vi "RFID_Barcode_Get.vi"(8 "error in (no error)":errorcluster, 11 "Ref in":T1={"MS SQL Connection"=refnum, "UDL File"=path "", "Time"="", "DCODE"="", "WIP+1"=0, "MC No?"=0, "POKAYOKE?"=FALSE, "Expected Result"="", "Result [Status]"="", "Clock"=0.0, "RFID"="", "WIP Queue"=refnum, "TS Parameter"={"ProfitCenterCode"="", "LineCode"="", "WorkOrderNumber"="", "Model"="", "Model_with_Prefix"="", "VendorCode"="", "SetParameterDateCode"="", "PokaYoke"=0, "Target"=1, "Live_DateCode"="", "CustomerPartNumber"="", "Hand"="", "Ent_Stamp"=timestamp(0 s since 1904-01-01), "STS_CD"=0.0}, "Data_Queue"=[], "RFID Serial No."=""} {"TS Parameter"."Target" min=1 max=100000; "TS Parameter"."PokaYoke" min=0 max=1}) -> (0 "error out":errorcluster, 1 "Serial No":string, 2 "Expected Barcode":string, 3 "Ref out":T1={"MS SQL Connection"=refnum, "UDL File"=path "", "Time"="", "DCODE"="", "WIP+1"=0, "MC No?"=0, "POKAYOKE?"=FALSE, "Expected Result"="", "Result [Status]"="", "Clock"=0.0, "RFID"="", "WIP Queue"=refnum, "TS Parameter"={"ProfitCenterCode"="", "LineCode"="", "WorkOrderNumber"="", "Model"="", "Model_with_Prefix"="", "VendorCode"="", "SetParameterDateCode"="", "PokaYoke"=0, "Target"=1, "Live_DateCode"="", "CustomerPartNumber"="", "Hand"="", "Ent_Stamp"=timestamp(0 s since 1904-01-01), "STS_CD"=0.0}, "Data_Queue"=[], "RFID Serial No."=""} {"TS Parameter"."Target" min=1 max=100000; "TS Parameter"."PokaYoke" min=0 max=1})   [LabVIEW 2020]
uses:
  Controls/TD SQL.ctl
  <vilib>/addons/database/Connection.llb/Conn ObjectReference.ctl
  Controls/WIP_State.ctl
  Controls/TS_Parameter.ctl
  <vilib>/addons/database/NI_Database_API.lvlib
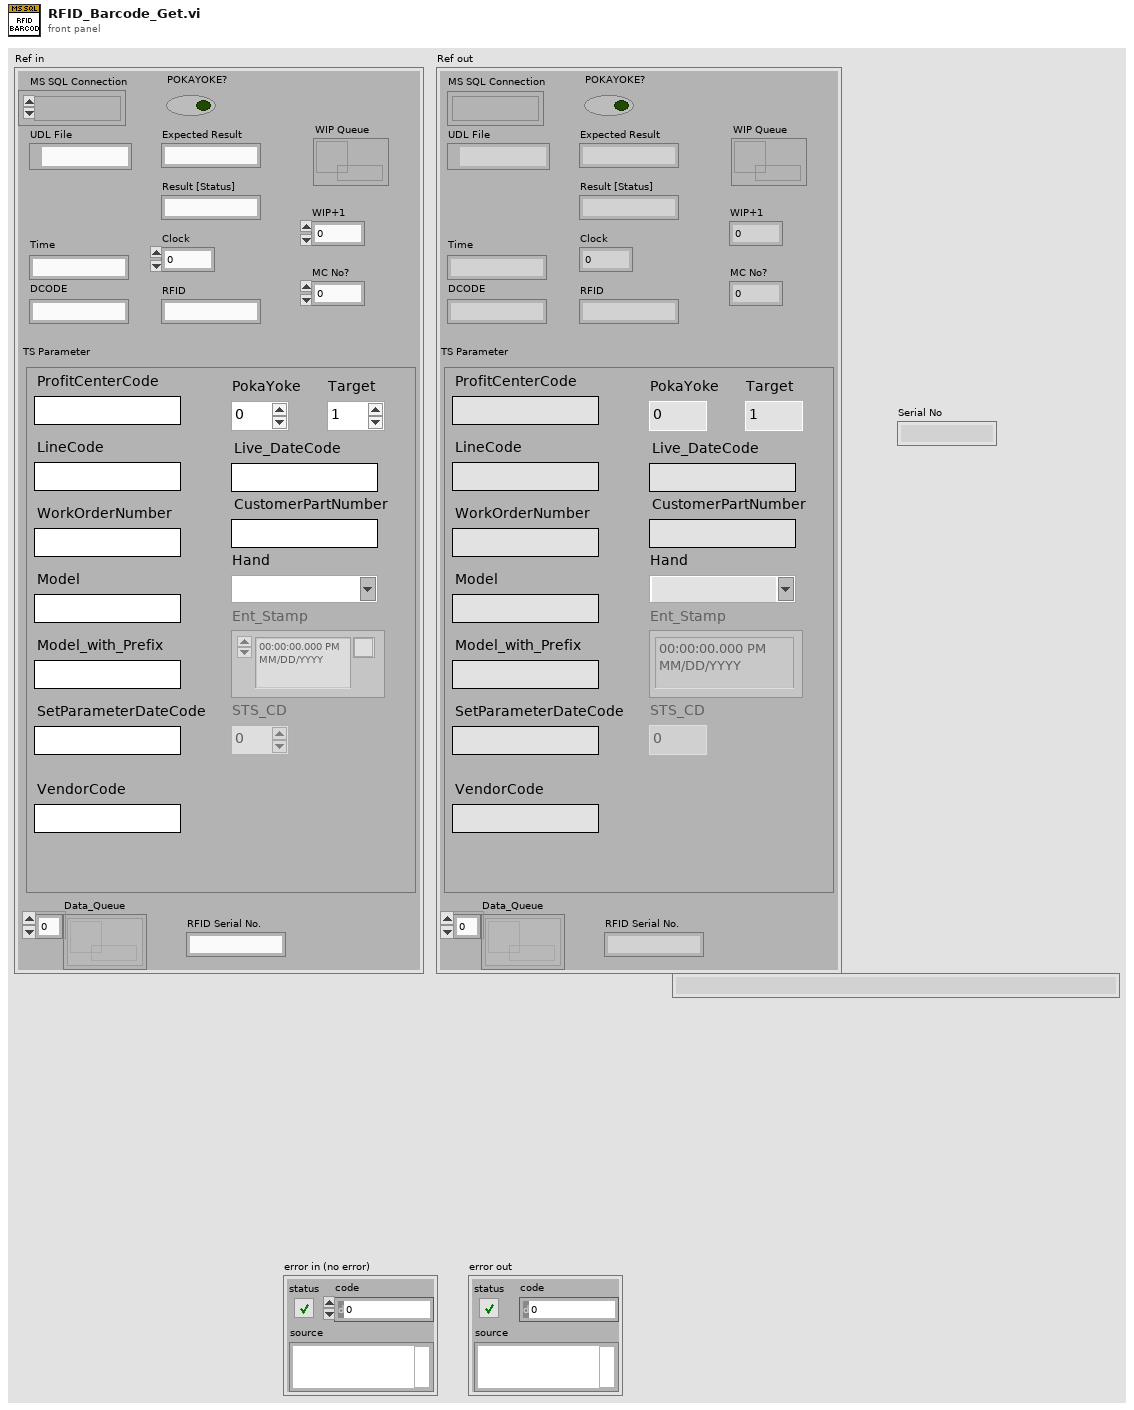
[diagram p1: front panel]
types:
  T1 = typedef "TD SQL.ctl" = cluster{"MS SQL Connection":T2, "UDL File":path, "Time":string, "DCODE":string, "WIP+1":i64, "MC No?":i32, "POKAYOKE?":bool, "Expected Result":string, "Result [Status]":string, "Clock":dbl, "RFID":string, "WIP Queue":refnum<queue>, "TS Parameter":T3, "Data_Queue":refnum<queue>[], "RFID Serial No.":string}
  T2 = typedef "NI_Database_API.lvlib/Conn ObjectReference.ctl" = refnum<k1>
  T3 = typedef "TS_Parameter.ctl" = cluster{"ProfitCenterCode":string, "LineCode":string, "WorkOrderNumber":string, "Model":string, "Model_with_Prefix":string, "VendorCode":string, "SetParameterDateCode":string, "PokaYoke":i32, "Target":i32, "Live_DateCode":string, "CustomerPartNumber":string, "Hand":string, "Ent_Stamp":timestamp, "STS_CD":dbl}
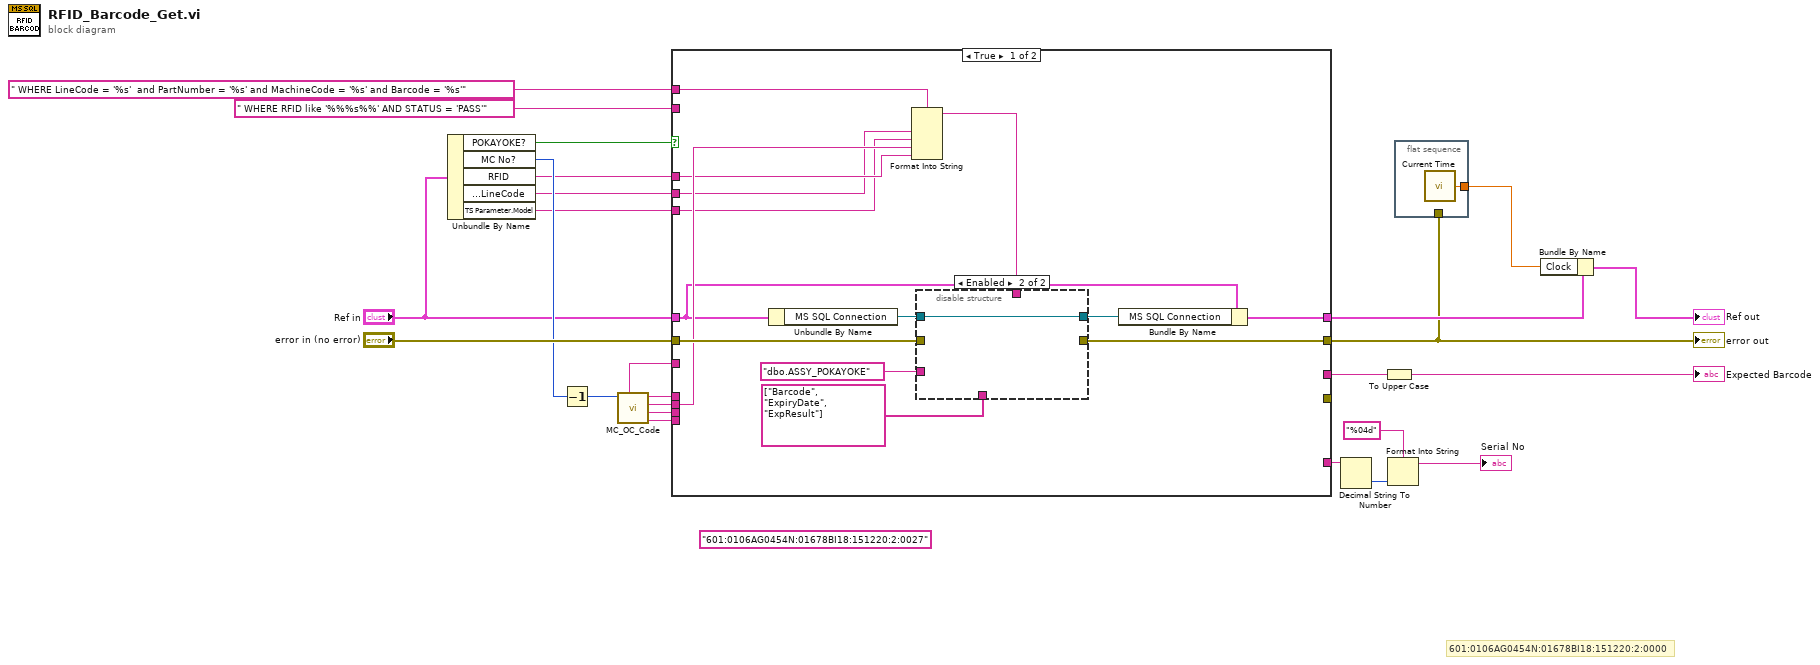
[diagram p0: block diagram]
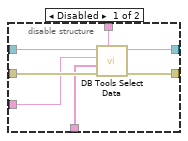
[diagram p2: hidden frame]
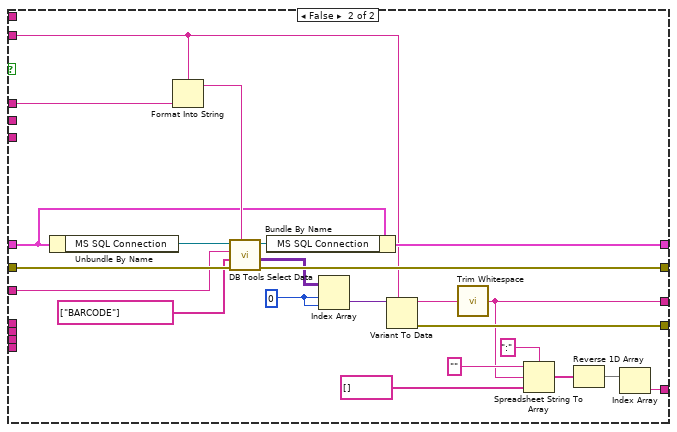
[diagram p3: hidden frame]
diagram:
  (unwired) "601:0106AG0454N:01678BI18:151220:2:0027" ("Expected Result")
  # "601:0106AG0454N:01678BI18:151220:2:0000"
  n1 = Unbundle By Name("Ref in") -> ("POKAYOKE?"=w16:bool, "MC No?"=w17:i32, "RFID"=w10:string, "TS Parameter.LineCode"=w2:string, "TS Parameter.Model"=w1:string)
  n2 = Decrement(x=w17) -> (x-1=w8:i32)
  n3 = call "MC_OC_Code.vi"("index"=w8) -> ("Code Query"=w22:string, "TS CODE TAG"=w19:string, "Machine Code"=w23:string, "Operation Code"=w24:string, "Table Name"=w18:string)  [unwired: 4 in, 2 out]
  n4 = case shown="True" w16 {
    tunnel: [w39 w70] -> w20
    tunnel: [w38 w63] -> w11
    tunnel: "error in (no error)" -> [w36 w69]
    tunnel: w10 -> [w31 w67]
    tunnel: "Ref in" -> [w28 w61]
    tunnel: w22 -> [_ _]
    tunnel: w23 -> [w32 _]
    tunnel: w24 -> [_ _]
    tunnel: w18 -> [_ w65]
    tunnel: [_ w50] -> w13
    tunnel: " WHERE LineCode = '%s'  and PartNumber = '%s' and MachineCode = '%s' and Barcode = '%s'" -> [w30 _]
    tunnel: w19 -> [_ _]
    tunnel: [_ w57] -> _
    tunnel: [_ w51] -> w5
    tunnel: " WHERE RFID like '%%%s%%' AND STATUS = 'PASS'" -> [_ w48]
    tunnel: w2 -> [w27 _]
    tunnel: w1 -> [w26 _]
    frame True {
      n5 = Unbundle By Name(w28) -> ("MS SQL Connection"=w35:T2)
      n6 = Format Into String(format string=w30, w27, w26, w32, w31) -> (resulting string=w34:string)  [unwired: 2 in, 1 out]
      n7 = disable-structure shown="Enabled" {
        disable-tunnel: [w46 _] -> w38
        disable-tunnel: [w45 w47] -> w37
        disable-tunnel: w36 -> [w44 _]
        disable-tunnel: w35 -> [w43 w47]
        disable-tunnel: w34 -> [w42 _]
        disable-tunnel: string[] ["Barcode", "ExpiryDate", "ExpResult"] ("columns") -> [w41 _]
        disable-tunnel: "dbo.ASSY_POKAYOKE" -> [w40 _]
        frame Disabled {
          n8 = call <vilib>:"DB Tools Select Data.vi"("condition"=w42, "error in (no error)"=w44, "columns"=w41, "table"=w40, "connection reference"=w43) -> ("error out"=w46:errorcluster, "connection reference out"=w45:T2)  [unwired: 1 in, 1 out]
        }
        frame Enabled {
        }
      }
      n9 = Bundle By Name(cluster=w28, "MS SQL Connection"=w37) -> (w39:T1)
    }
    frame False {
      w59 = 0 ("index (row)")
      n10 = Unbundle By Name(w61) -> ("MS SQL Connection"=w68:T2)
      n11 = Format Into String(format string=w48, w67) -> (resulting string=w64:string)  [unwired: 2 in, 1 out]
      n12 = call <vilib>:"DB Tools Select Data.vi"("condition"=w64, "error in (no error)"=w69, "columns"=string[] ["BARCODE"], "table"=w65, "connection reference"=w68) -> ("error out"=w63:errorcluster, "data"=w60:variant[][], "connection reference out"=w62:T2)  [unwired: 1 in]
      n13 = Bundle By Name(cluster=w61, "MS SQL Connection"=w62) -> (w70:T1)
      n14 = Index Array(array=w60, index (row)=w59, index (col)=w59) -> (element=w58:variant)
      n15 = Variant To Data(type=w48, Variant=w58) -> (data=w49:string, error out=w57:errorcluster)  [unwired: 1 in]
      n16 = call <vilib>:"Trim Whitespace.vi"("string"=w49) -> ("trimmed string"=w50:string)  [unwired: 1 in]
      n17 = Spreadsheet String To Array(delimiter (Tab)=":", format string="", spreadsheet string=w50, array type (2D Dbl)=string[] []) -> (array=w53:string[])
      n18 = Reverse 1D Array(array=w53) -> (reversed array=w52:string[])
      n19 = Index Array(array=w52) -> (element=w51:string)  [unwired: 1 in]
    }
  }
  "error out" <- w11
  n20 = Decimal String To Number(string=w5) -> (number=w6:i32)  [unwired: 2 in, 1 out]
  n21 = To Upper Case(1:w13) -> (0:→"Expected Barcode":string)
  n22 = Format Into String(format string="%04d", w6) -> (resulting string=→"Serial No":string)  [unwired: 2 in, 1 out]
  n23 = flat-sequence {
    tunnel: [w71] -> w12
    tunnel: w11 -> [_]
    frame #0 {
      n24 = call <userlib>:"Current Time.vi"() -> ("Current Time (Sec)"=w71:dbl)  [unwired: 15 in]
    }
  }
  n25 = Bundle By Name(cluster=w20, "Clock"=w12) -> (→"Ref out":T1)
